vi "RegiMedic.vi"() -> ()   [LabVIEW 2021]
uses:
  Control 1.ctl
  <vilib>/Utility/NIReport.llb/Report Type.ctl
  <vilib>/Utility/NIReport.llb/Append Report Text (str wrap).vi
  <vilib>/Utility/NIReport.llb/Append Text Table to Report (wrap).vi
  <vilib>/Utility/NIReport.llb/NI_report.lvclass
  <vilib>/Utility/NIReport.llb/NI_ReportGenerationCore.lvlib
panel:
  in  "Enviar":bool
  out "Estado":bool
  in  "Sensor Tx":bool
  in  "report file path":path
  in  "stop":bool
  in  "CONSUMO DE MEDICAMENTOS":T1
  # "PANEL DE REGISTRO DE MEDICAMENTOS"
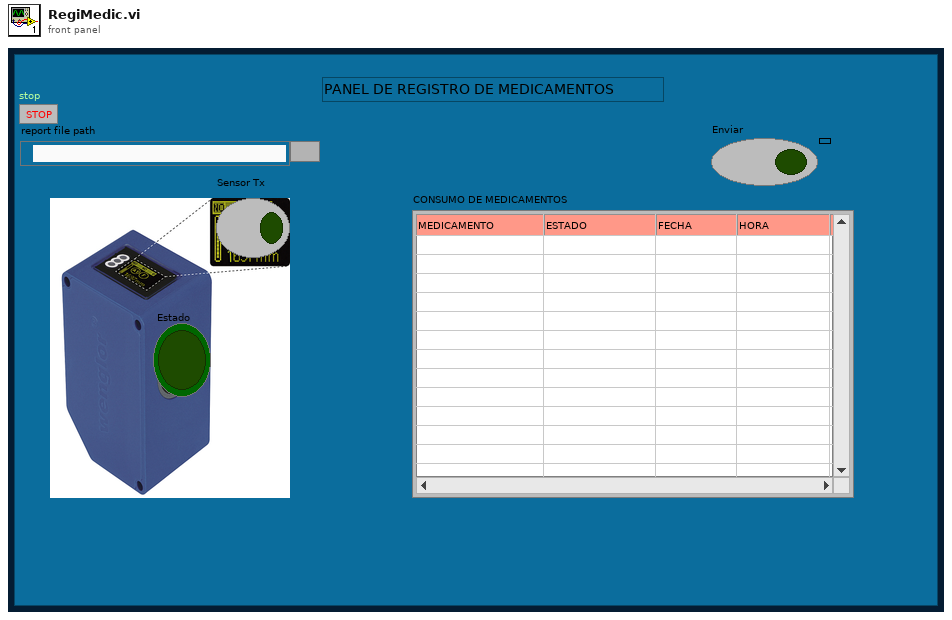
[diagram p1: front panel]
types:
  T1 = typedef "Control 1.ctl" = string[][]
  T2 = typedef "NI_ReportGenerationCore.lvlib/Report Type.ctl" = enum16{"HTML", "Word", "Excel"}
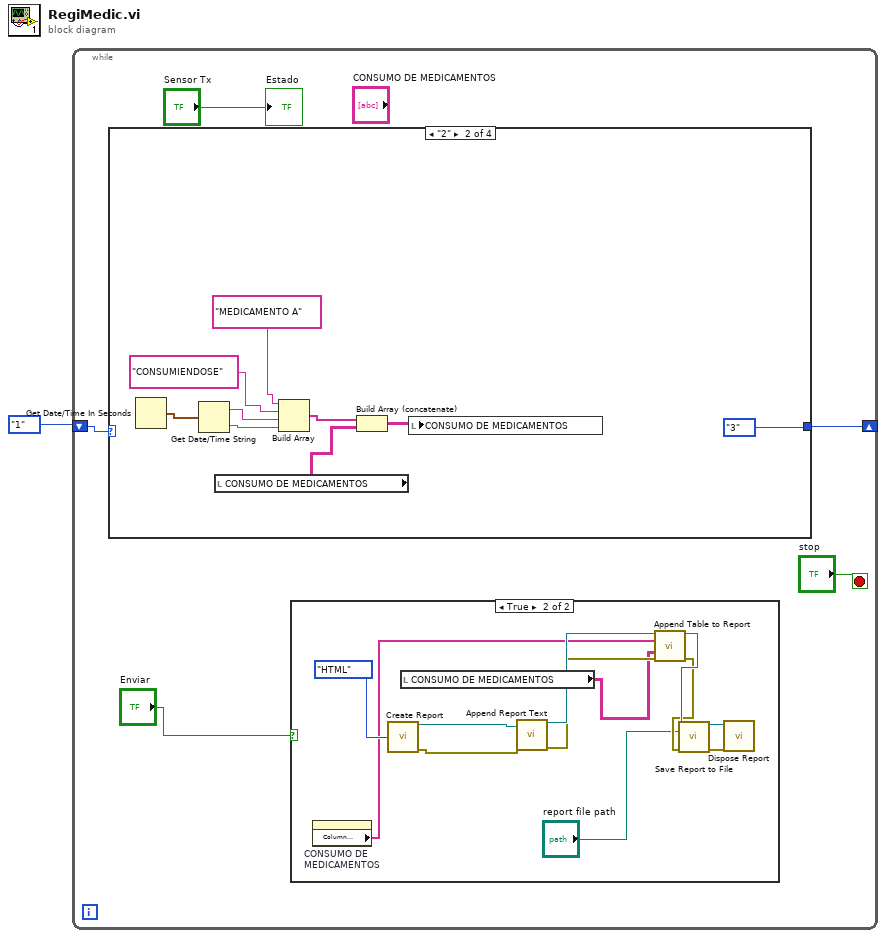
[diagram p0: block diagram]
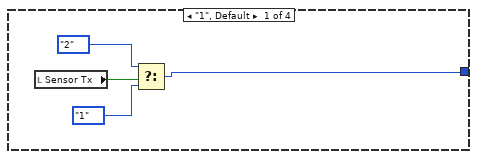
[diagram p3: hidden frame]
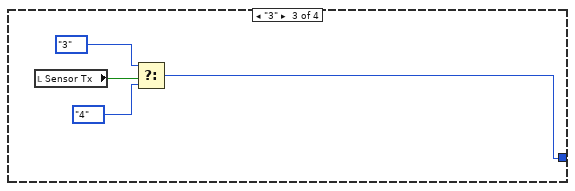
[diagram p4: hidden frame]
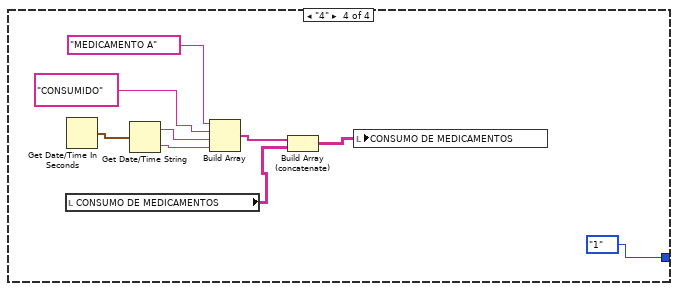
[diagram p5: hidden frame]
diagram:
  n1 = while {
    shift-right: [w3] -> _
    shift-left: enum16{"1", "2", "3", "4", "5", "6"}."1" -> [w4]
    stop <- "stop" stop-if-true
    n2 = case shown="\"2\"" w4 {
      tunnel: [w19 enum16{"1", "2", "3", "4", "5", "6"}."3" w32 enum16{"1", "2", "3", "4", "5", "6"}."1"] -> w3
      frame "1", Default {
        n3 = local read "Sensor Tx"() -> (w22:bool)
        n4 = Select(t=enum16{"1", "2", "3", "4", "5", "6"}."2", s=w22, f=enum16{"1", "2", "3", "4", "5", "6"}."1") -> (s? t:f=w19:enum16{"1", "2", "3", "4", "5", "6"})
      }
      frame "2" {
        n5 = Get Date/Time In Seconds() -> (seconds since 1Jan1904=w28:timestamp)
        n6 = Get Date/Time String(seconds (now)=w28) -> (date string=w26:string, time string=w27:string)  [unwired: 2 in]
        n7 = local read "CONSUMO DE MEDICAMENTOS"() -> (w29:T1)
        n8 = Build Array("MEDICAMENTO A" ("element"), "CONSUMIENDOSE" ("element"), w26, w27) -> (w31:string[])
        n9 = Build Array (concatenate)(w31, w29) -> (w30:T1)
        n10 = local write "CONSUMO DE MEDICAMENTOS"(w30) -> ()
      }
      frame "3" {
        n11 = local read "Sensor Tx"() -> (w35:bool)
        n12 = Select(t=enum16{"1", "2", "3", "4", "5", "6"}."3", s=w35, f=enum16{"1", "2", "3", "4", "5", "6"}."4") -> (s? t:f=w32:enum16{"1", "2", "3", "4", "5", "6"})
      }
      frame "4" {
        n13 = local read "CONSUMO DE MEDICAMENTOS"() -> (w38:T1)
        n14 = Get Date/Time In Seconds() -> (seconds since 1Jan1904=w43:timestamp)
        n15 = Get Date/Time String(seconds (now)=w43) -> (date string=w41:string, time string=w42:string)  [unwired: 2 in]
        n16 = Build Array("MEDICAMENTO A" ("element"), "CONSUMIDO" ("element"), w41, w42) -> (w44:string[])
        n17 = Build Array (concatenate)(w44, w38) -> (w37:T1)
        n18 = local write "CONSUMO DE MEDICAMENTOS"(w37) -> ()
      }
    }
    n19 = case shown="True" "Enviar" {
      frame False {
      }
      frame True {
        n20 = property on="CONSUMO DE MEDICAMENTOS" class="Tbl (strict)"() -> ("Column Headers[]"=w7:string[])  [unwired: 2 in, 2 out]
        n21 = call <vilib>:"Create Report.vi"("report type"=Report_Type."HTML") -> ("report out"=w11:refnum<class "NI_report.lvclass">, "error out"=w10:errorcluster)  [unwired: 13 in]
        n22 = local read "CONSUMO DE MEDICAMENTOS"() -> (w8:T1)
        n23 = call-poly <vilib>:"Append Report Text.vi"("report in"=w11, "error in (no error)"=w10) -> ("report out"=w17:refnum<class "NI_report.lvclass">, "error out"=w16:errorcluster)  [unwired: 10 in, 2 out]
        n24 = call-poly <vilib>:"Append Table to Report.vi"("report in"=w17, "column headers"=w7, "text data"=w8, "error in (no error)"=w16) -> ("report out"=w15:refnum<class "NI_report.lvclass">, "error out"=w14:errorcluster)  [unwired: 8 in, 2 out]
        n25 = call-dynamic "Save Report to File.vi"("report in"=w15, "report file path"="report file path", "error in (no error)"=w14) -> ("report out"=w13:refnum<class "NI_report.lvclass">, "error out"=w12:errorcluster)  [unwired: 11 in]
        n26 = call-dynamic "Dispose Report.vi"("report in"=w13, "error in (no error)"=w12) -> ()  [unwired: 13 in, 1 out]
      }
    }
    "Estado" <- "Sensor Tx"
  }
